vi "DefensePsSkill.vi"(9 "Game in":refnum<class "Game.lvclass">, 10 "Robot":refnum<class "Robot.lvclass">, 11 "DefensePsSkill in":refnum<class "DefensePsSkill.lvclass">) -> (2 "Robot out":refnum<class "Robot.lvclass">, 3 "DefensePsSkill out":refnum<class "DefensePsSkill.lvclass">)   [LabVIEW 2020, in "DefensePsSkill.lvclass"]
uses:
  DefensePsSkill.lvclass
  Robot_class/Robot.lvclass
  C:/Users/Pedro/Dropbox/My PC (LAPTOP-06JBDO7V)/Documents/GitHub/SSL_AI/Object_class/Object.lvclass
  Game_class/Game.lvclass
  Game_class/Game.lvclass/Game.ctl
  Object_class/Object.lvclass/Object.ctl
  Robot_class/Robot.lvclass/Robot.ctl
  Robot_class/Write dest_y.vi
  Object_class/Read y.vi
  Game_class/Read BallRef.vi
  Game_class/Read FieldRef.vi
  Object_class/Read x.vi
  Robot_class/Write dest_x.vi
  Robot_class/Write dest_orientation.vi
  Ball_class/Ball.lvclass
  Field_class/Field.lvclass
panel:
  out "error out 2":errorcluster
  in  "error in (no error) 2":errorcluster
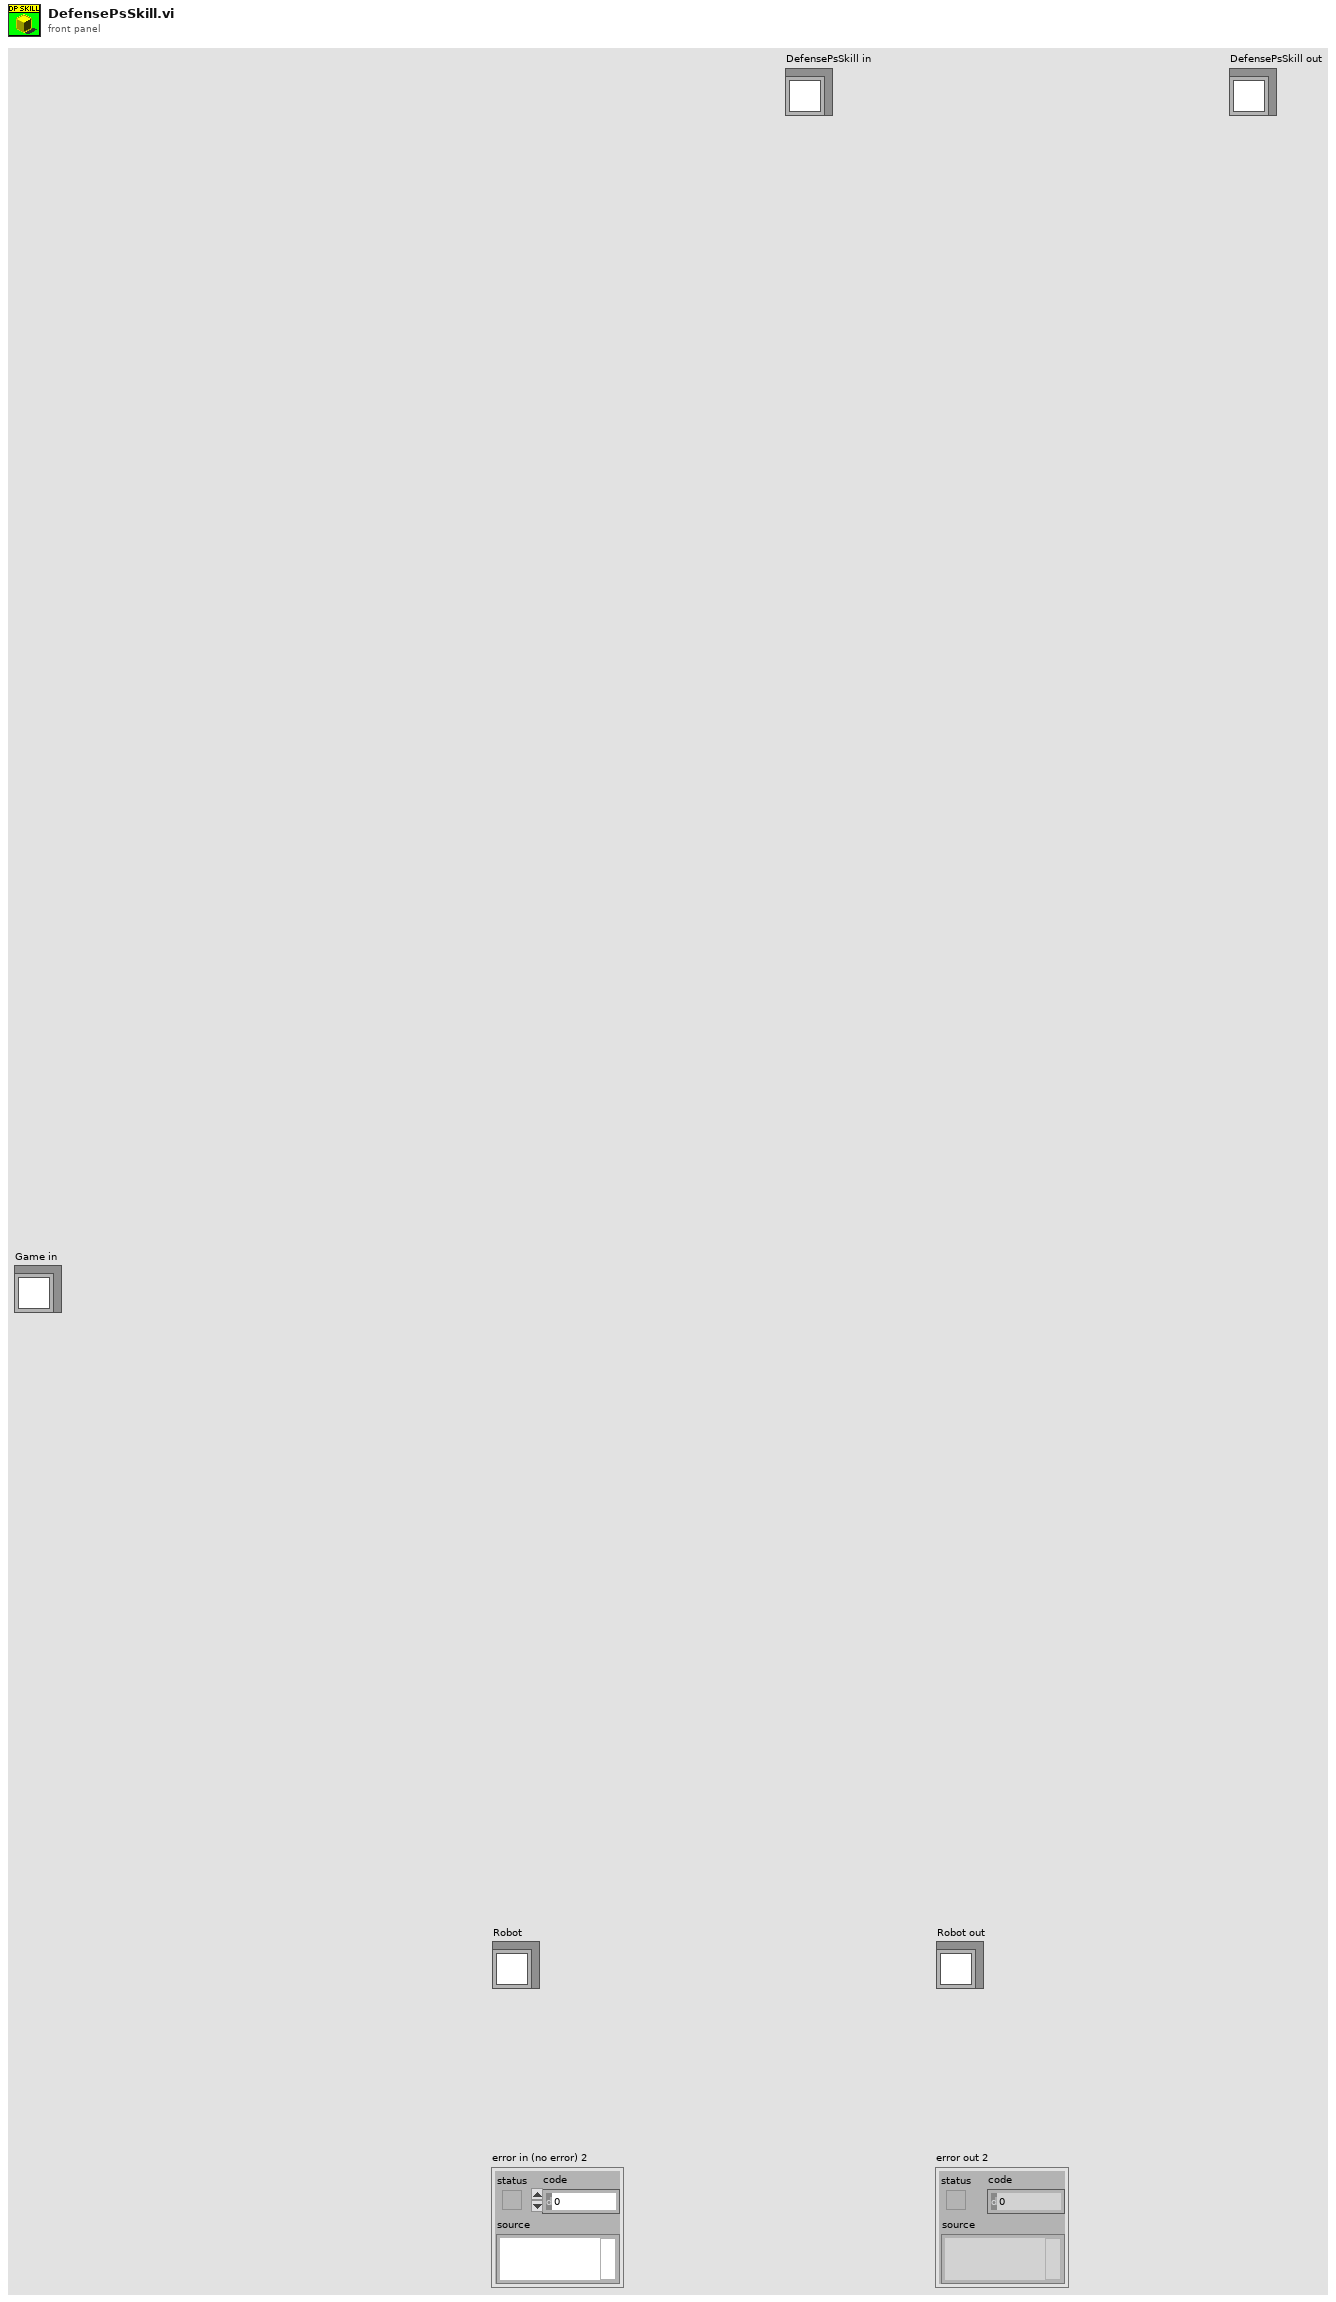
[diagram p1: front panel]
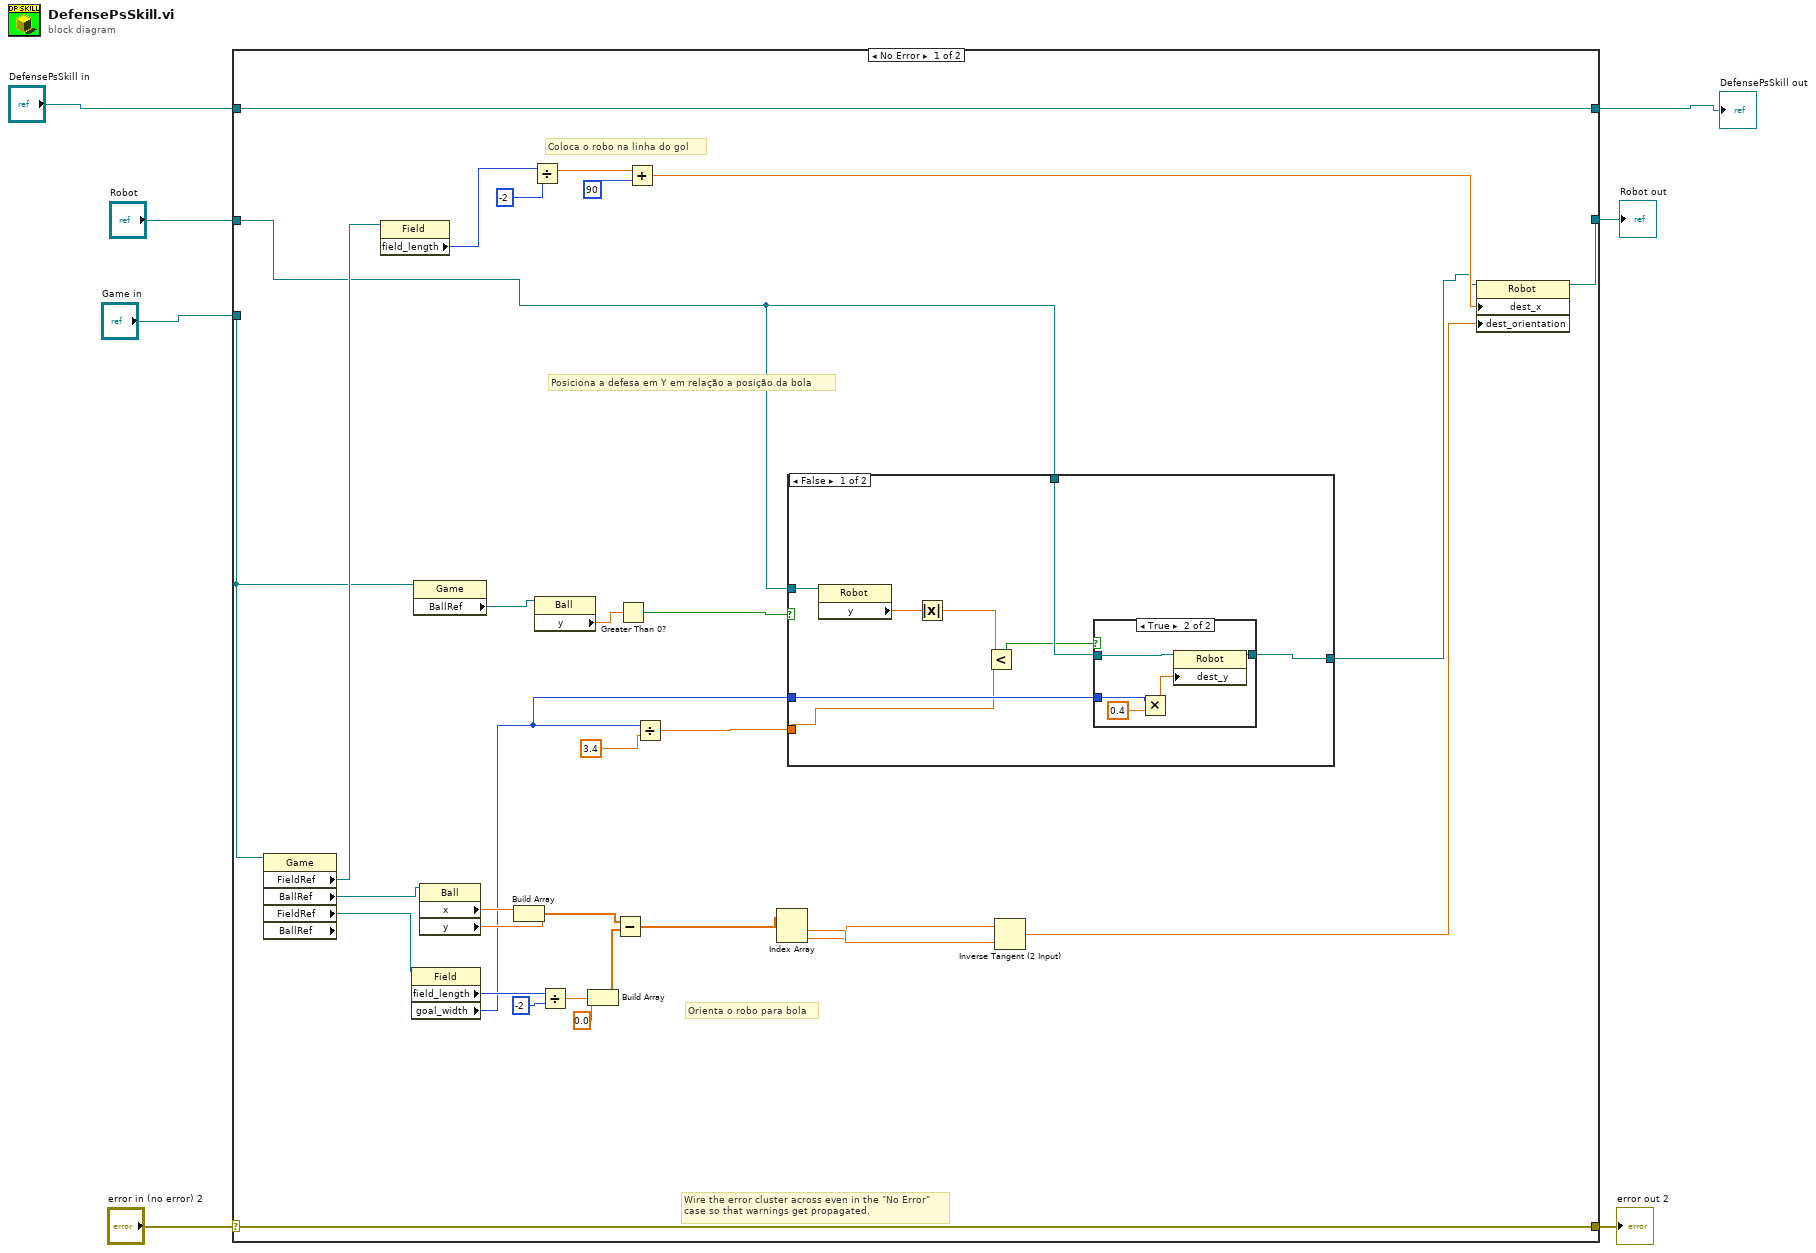
[diagram p0: block diagram]
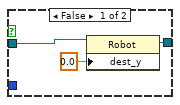
[diagram p2: hidden frame]
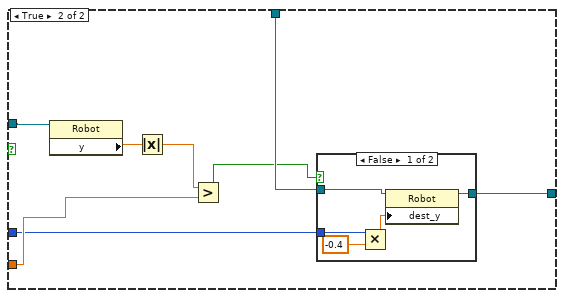
[diagram p3: hidden frame]
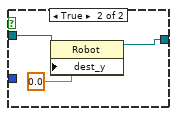
[diagram p4: hidden frame]
diagram:
  n1 = case shown="No Error" "error in (no error) 2" {
    selector: "error in (no error) 2" -> [w38 w74]
    tunnel: [w38 w74] -> w6
    tunnel: [w39 w73] -> w2
    tunnel: "DefensePsSkill in" -> [w39 w73]
    tunnel: "Robot" -> [w8 w72]
    tunnel: [w37 w72] -> w4
    tunnel: "Game in" -> [w11 _]
    frame No Error {
      # "Coloca o robo na linha do gol"
      # "Orienta o robo para bola"
      # "Posiciona a defesa em Y em relação a posição da bola"
      # "Wire the error cluster across even in the \"No Error\"\ncase so that warnings get propagated."
      n2 = property class="Game" props=["FieldRef", "BallRef", "FieldRef", "BallRef"](reference=w11) -> ("FieldRef"=w36:refnum<class "Field.lvclass">, "BallRef"=w31:refnum<class "Ball.lvclass">, "FieldRef"=w28:refnum<class "Field.lvclass">)  [unwired: 1 in, 3 out]
      n3 = property class="Field"(reference=w36) -> ("field_length"=w33:i32)  [unwired: 1 in, 2 out]
      n4 = property class="Field"(reference=w28) -> ("field_length"=w27:i32, "goal_width"=w13:i32)  [unwired: 1 in, 2 out]
      n5 = property class="Game"(reference=w11) -> ("BallRef"=w10:refnum<class "Ball.lvclass">)  [unwired: 1 in, 2 out]
      n6 = property class="Ball"(reference=w31) -> ("x"=w30:dbl, "y"=w29:dbl)  [unwired: 1 in, 2 out]
      n7 = Build Array(w30, w29) -> (w23:dbl[])
      n8 = Divide(x=w33, y=-2) -> (x/y=w32:dbl)
      n9 = property class="Ball"(reference=w10) -> ("y"=w9:dbl)  [unwired: 1 in, 2 out]
      n10 = Divide(x=w27, y=-2) -> (x/y=w25:dbl)
      n11 = Build Array(w25, 0.0 ("element")) -> (w22:dbl[])
      n12 = Subtract(x=w23, y=w22) -> (x-y=w21:dbl[])
      n13 = Greater Than 0?(x=w9) -> (x > 0?=w15:bool)
      n14 = Add(x=w32, y=90) -> (x+y=w17:dbl)
      n15 = Divide(x=w13, y=3.4) -> (x/y=w16:dbl)
      n16 = Index Array(array=w21) -> (element #1=w20:dbl, element #2=w19:dbl)  [unwired: 2 in]
      n17 = case shown="False" w15 {
        tunnel: w16 -> [w40 w62]
        tunnel: w8 -> [w47 w63]
        tunnel: [w45 w60] -> w14
        tunnel: w13 -> [w44 w59]
        tunnel: w8 -> [w41 w56]
        frame False {
          n18 = property class="Robot"(reference=w41) -> ("y"=w43:dbl)  [unwired: 1 in, 2 out]
          n19 = Absolute Value(x=w43) -> (abs(x)=w42:dbl)
          n20 = Less?(x=w42, y=w40) -> (x < y?=w46:bool)
          n21 = case shown="True" w46 {
            tunnel: w47 -> [w50 w53]
            tunnel: [w48 w52] -> w45
            tunnel: w44 -> [_ w51]
            frame False {
              n22 = property class="Robot"(reference=w50, "dest_y"=0.0) -> (reference out=w48:refnum<class "Robot.lvclass">)  [unwired: 1 in, 1 out]
            }
            frame True {
              n23 = Multiply(x=w51, y=0.4) -> (x*y=w54:dbl)
              n24 = property class="Robot"(reference=w53, "dest_y"=w54) -> (reference out=w52:refnum<class "Robot.lvclass">)  [unwired: 1 in, 1 out]
            }
          }
        }
        frame True {
          n25 = property class="Robot"(reference=w56) -> ("y"=w58:dbl)  [unwired: 1 in, 2 out]
          n26 = Absolute Value(x=w58) -> (abs(x)=w57:dbl)
          n27 = Greater?(x=w57, y=w62) -> (0:w61:bool)
          n28 = case shown="False" w61 {
            tunnel: w63 -> [w66 w71]
            tunnel: [w65 w69] -> w60
            tunnel: w59 -> [w64 _]
            frame False {
              n29 = Multiply(x=w64, y=-0.4) -> (x*y=w67:dbl)
              n30 = property class="Robot"(reference=w66, "dest_y"=w67) -> (reference out=w65:refnum<class "Robot.lvclass">)  [unwired: 1 in, 1 out]
            }
            frame True {
              n31 = property class="Robot"(reference=w71, "dest_y"=0.0) -> (reference out=w69:refnum<class "Robot.lvclass">)  [unwired: 1 in, 1 out]
            }
          }
        }
      }
      n32 = Inverse Tangent (2 Input)(1:w20, 2:w19) -> (0:w18:dbl)
      n33 = property class="Robot"(reference=w14, "dest_x"=w17, "dest_orientation"=w18) -> (reference out=w37:refnum<class "Robot.lvclass">)  [unwired: 1 in, 1 out]
    }
    frame Error {
    }
  }
  "DefensePsSkill out" <- w2
  "error out 2" <- w6
  "Robot out" <- w4
